vi "_Test_VC_Unit_test.vi"() -> ()   [LabVIEW 2023]
uses:
  RDB/RDB.lvlib
panel:
  out "error out 2":errorcluster
  out "error out":errorcluster
  out "simFrame":dbl
  out "simTime":dbl
  out "Array 2":u8[](array[numeric])
  out "Array":string[](array[string])
  in  "file path (use dialog)":path=path "\\\\10.144.128.67\\adas_nas/VTD/testData/debug_TCmsg"
  in  "path in":path=path "C:/dev/Hexagon-VTD-Custom-Device/Libraries/libVC.dll"
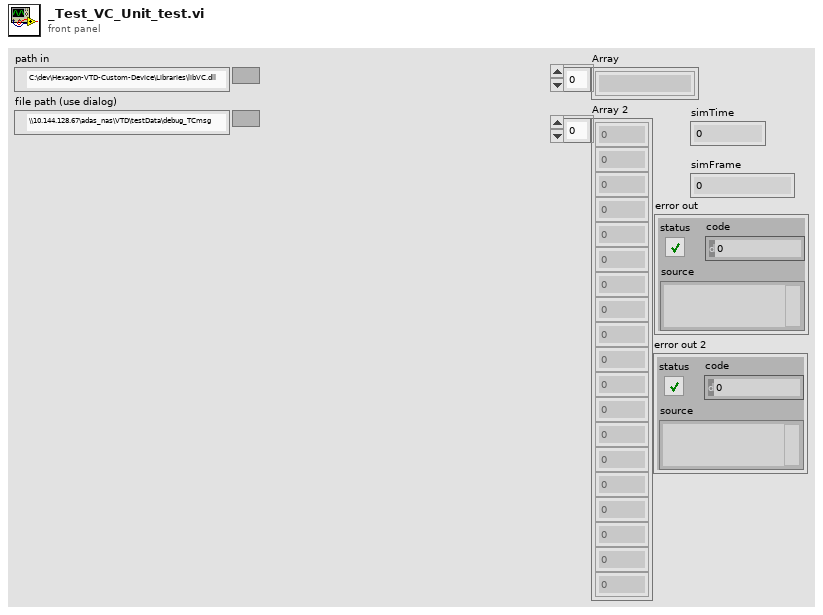
[diagram p1: front panel]
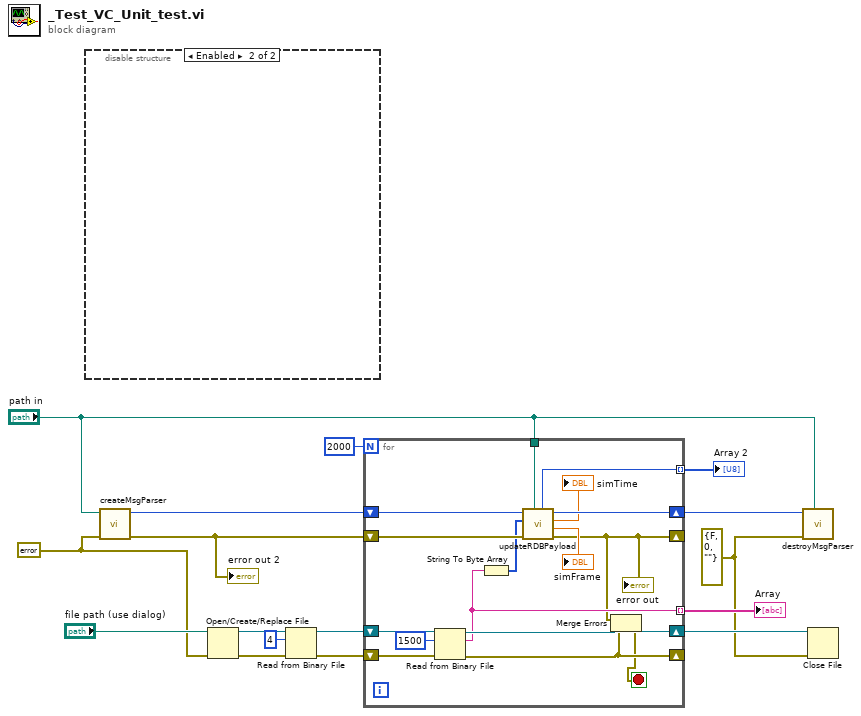
[diagram p0: block diagram]
diagram:
  w6 = errorcluster {"status"=FALSE, "code"=0, "source"=""} ("error in (no error)")
  w9 = errorcluster {"status"=FALSE, "code"=0, "source"=""} ("error in (no error)")
  n1 = disable-structure shown="Enabled" {
    frame Disabled {
    }
    frame Enabled {
    }
  }
  n2 = call "createMsgParser.vi"("error in (no error)"=w9, "path in"="path in") -> ("error out"=w10:errorcluster, "paeseHandle"=w11:u64)  [unwired: 8 in]
  "error out 2" <- w10
  n3 = Open/Create/Replace File(file path (use dialog)="file path (use dialog)", error in=w9) -> (refnum out=w5:refnum<file>, error out=w3:errorcluster)  [unwired: 4 in, 1 out]
  n4 = Read from Binary File(8:w3, 10:4 ("count (1)"), 11:w5) -> (0:w2:errorcluster, 3:w4:refnum<file>)  [unwired: 3 in, 2 out]
  n5 = for {
    N: 2000 -> [_]
    tunnel: "path in" -> [w29]
    shift-right: [w30] -> w7
    shift-left: w11 -> [w32]
    shift-right: [w19] -> _
    shift-left: w10 -> [w31]
    shift-right: [w26] -> w16
    shift-left: w4 -> [w28]
    shift-right: [w18] -> _
    shift-left: w2 -> [w27]
    tunnel: [w23] -> w14 mode=indexing
    tunnel: [w22] -> w13 mode=indexing
    stop <- w17 stop-if-true
    n6 = Read from Binary File(8:w27, 10:1500 ("count (1)"), 11:w28) -> (0:w18:errorcluster, 2:w23:string, 3:w26:refnum<file>)  [unwired: 3 in, 1 out]
    n7 = String To Byte Array(string=w23) -> (unsigned byte array=w24:u8[])
    n8 = call "updateRDBPayload.vi"("path in"=w29, "error in (no error)"=w31, "payload"=w24, "paeseHandle in"=w32) -> ("error out"=w19:errorcluster, "simFrame"=→"simFrame":dbl, "simTime"=→"simTime":dbl, "paeseHandle out"=w30:u64, "isComplete"=w22:u8)  [unwired: 3 in]
    "error out" <- w19
    n9 = Merge Errors(w19, w18) -> (w17:errorcluster)
  }
  "Array" <- w14
  "Array 2" <- w13
  n10 = call "destroyMsgParser.vi"("path in"="path in", "error in (no error)"=w6, "parserHandle"=w7) -> ()  [unwired: 8 in, 1 out]
  n11 = Close File(refnum=w16, error in=w6) -> ()  [unwired: 2 out]
